vi "FTP.vi"(8 "error in (no error)":errorcluster caption="错误输入（无错误）", 10 "远程路径":string, 11 "local path":path caption="文件路径") -> (0 "error out":errorcluster caption="错误输出")   [LabVIEW 2020]
uses:
  <vilib>/FTP/NI_FTP.lvlib
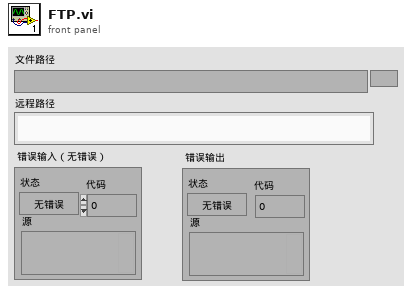
[diagram p1: front panel]
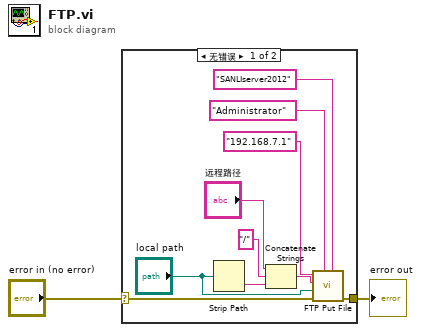
[diagram p0: block diagram]
diagram:
  n1 = case shown="无错误" "error in (no error)" {
    selector: "error in (no error)" -> [w3 w13]
    tunnel: [w4 w13] -> w2
    frame No Error {
      n2 = Strip Path(path="local path") -> (name=w7:string)  [unwired: 1 out]
      n3 = Concatenate Strings("远程路径", "/" ("字符串"), w7) -> (w8:string)
      n4 = call <vilib>:"FTP Put File.vi"("password"="SANLIserver2012", "user"="Administrator", "error in (no error)"=w3, "local path"="local path", "remote path"=w8, "host"="192.168.7.1") -> ("error out"=w4:errorcluster)  [unwired: 4 in, 1 out]
    }
    frame Error {
    }
  }
  "error out" <- w2
